vi "GetUpcomingComics.vi"(8 "error in":errorcluster) -> (0 "error out":errorcluster)   [LabVIEW 2024]
uses:
  <vilib>/addons/_JKI.lib/REST Client/classes/REST Client/REST Client.lvclass
panel:
  in  "Months Ahead":i32=3
  in  "Stop":bool
  out "last offset":i32
  out "progress":i32(slide) caption="200 of 203" scale=0.0..203.0
  # "Run Organize New comics after running this guy"
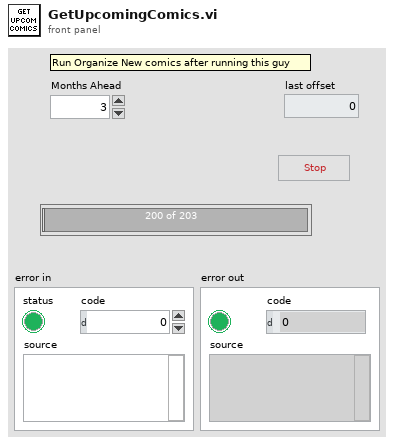
[diagram p1: front panel]
types:
  T1 = typedef "comics.reply--cluster.ctl" = cluster{"code":i32, "status":string, "etag":string, "data":cluster{"offset":i32, "limit":i32, "total":i32, "count":i32, "results":T2[]}}
  T2 = typedef "comic--cluster.ctl" = cluster{"id":i32, "digitalId":i32, "title":string, "issueNumber":i32, "variantDescription":string, "description":string, "modified":variant, "upc":string, "format":string, "pageCount":i32, "resourceURI":string, "urls":cluster{"type":string, "url":string}[], "series":cluster{"resourceURI":string, "name":string}, "dates":cluster{"type":string, "date":string}[], "prices":cluster{"price":dbl, "type":string}[], "thumbnail":cluster{"path":string, "extension":string}, "images":cluster{"path":string, "extension":string}[], "creators":cluster{"available":i32, "returned":i32, "collectionURI":string, "items":cluster{"resourceURI":string, "name":string, "role":string}[]}, "characters":cluster{"available":i32, "returned":i32, "collectionURI":string, "items":cluster{"resourceURI":string, "name":string}[]}, "stories":cluster{"available":i32, "returned":i32, "collectionURI":string, "items":cluster{"resourceURI":string, "name":string, "type":string}[]}, "events":cluster{"available":i32, "returned":i32, "collectionURI":string, "items":cluster{"resourceURI":string, "name":string}[]}}
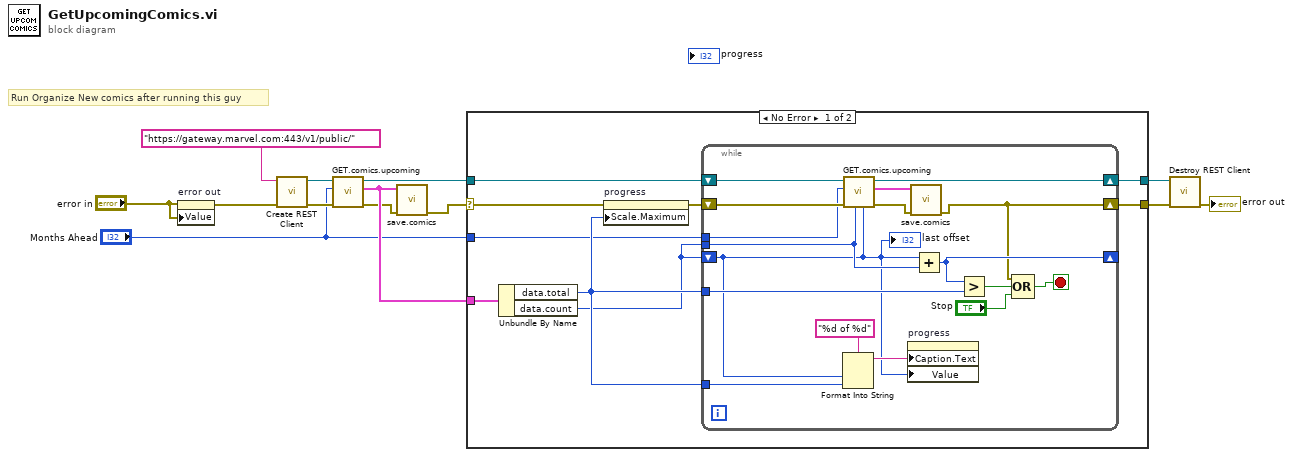
[diagram p0: block diagram]
diagram:
  # "Run Organize New comics after running this guy"
  n1 = property on="error out" class="Clust (strict)"(error in="error in", "Value"="error in") -> (error out=w8:errorcluster)  [unwired: 1 in, 1 out]
  n2 = call <vilib>:"Create REST Client.vi"("error in (no error)"=w8, "Base URL"="https://gateway.marvel.com:443/v1/public/") -> ("error out"=w3:errorcluster, "REST Client out"=w4:refnum<class "REST Client.lvclass">)  [unwired: 8 in]
  n3 = call "GET.comics.upcoming.vi"("error in (no error)"=w3, "Months Ahead"="Months Ahead", "REST Client in"=w4) -> ("error out"=w2:errorcluster, "data"=w6:T1, "REST Client out"=w5:refnum<class "REST Client.lvclass">)  [unwired: 6 in]
  n4 = call "save.comics.vi"("error in"=w2, "data"=w6) -> ("error out"=w9:errorcluster)  [unwired: 9 in]
  n5 = case shown="No Error" w9 {
    selector: w9 -> [w16 w40]
    tunnel: w6 -> [w22 _]
    tunnel: w5 -> [w21 w41]
    tunnel: [w20 w41] -> w11
    tunnel: [w19 w40] -> w10
    tunnel: "Months Ahead" -> [w14 _]
    frame No Error {
      n6 = Unbundle By Name(w22) -> ("data.total"=w17:i32, "data.count"=w15:i32)
      n7 = property on="progress" class="Slide (strict)"(error in=w16, "Scale.Maximum"=w17) -> (error out=w18:errorcluster)  [unwired: 1 in, 1 out]
      n8 = while {
        shift-right: [w27] -> w20
        shift-left: w21 -> [w28]
        shift-right: [w36] -> w19
        shift-left: w18 -> [w26]
        tunnel: w15 -> [w25]
        shift-right: [w39] -> _
        shift-left: w15 -> [w24]
        tunnel: w17 -> [w38]
        tunnel: w17 -> [w33]
        tunnel: w14 -> [w23]
        stop <- w35 stop-if-true
        n9 = Format Into String(format string="%d of %d", w24, w33) -> (resulting string=w32:string)  [unwired: 2 in, 1 out]
        n10 = call "GET.comics.upcoming.vi"("series offset"=w24, "Number of Series to GET"=w25, "error in (no error)"=w26, "Months Ahead"=w23, "REST Client in"=w28) -> ("error out"=w30:errorcluster, "data"=w29:T1, "REST Client out"=w27:refnum<class "REST Client.lvclass">)  [unwired: 4 in]
        n11 = property on="progress" class="Slide (strict)"("Caption.Text"=w32, "Value"=w24) -> ()  [unwired: 2 in, 2 out]
        n12 = call "save.comics.vi"("error in"=w30, "data"=w29) -> ("error out"=w36:errorcluster)  [unwired: 9 in]
        n13 = Add(x=w24, y=w25) -> (x+y=w39:i32)
        n14 = Greater?(x=w39, y=w38) -> (0:w37:bool)
        n15 = Compound Arithmetic op=OR(w36, w37, "Stop") -> (w35:bool)
        "last offset" <- w24
      }
    }
    frame Error {
    }
  }
  n16 = call-dynamic "Destroy REST Client.vi"("error in (no error)"=w10, "REST Client in"=w11) -> ("error out"=→"error out":errorcluster)  [unwired: 9 in]
